vi "zad11.vi"() -> ()   [LabVIEW 2025]
uses:
  state.ctl
  coffee.ctl
  delay_control.ctl
panel:
  out "error out":errorcluster
  in  "error in":errorcluster
  in  "Stop":bool
  out "Whipped cream":bool
  out "Chocolate Syrup":bool
  out "Milk Foam":bool
  out "Steamed Milk":bool
  out "Espresso":bool
  in  "Cafe Mocha":bool
  in  "Cafe Latte":bool
  in  "Espresso Macchiato":bool
  in  "Espresso":bool
  # "Wybierz kawe:"
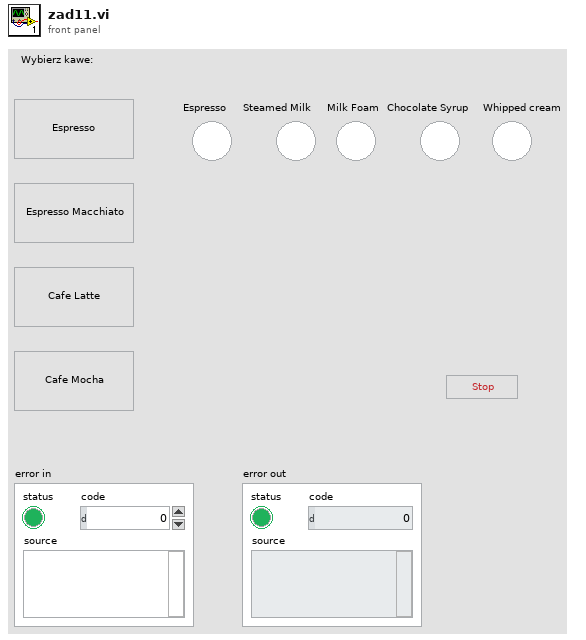
[diagram p1: front panel]
types:
  T1 = typedef "state.ctl" = enum16{"Init", "Idle", "espresso", "milk_foam", "steamed_milk", "whipped_cream", "chocolate_syrup", "save", "stop", "delay"}
  T2 = typedef "delay_control.ctl" = cluster{"time":dbl, "next state":T1}
  T3 = typedef "coffee.ctl" = cluster{"Type_Cof":string, "Cafe":enum16{"None", "espresso", "espresso macchiato", "caffe latte", "cafe mocha"}}
  T4 = enum16{"None", "espresso", "espresso macchiato", "caffe latte", "cafe mocha"}
  T5 = enum16{"open", "replace", "create", "open or create", "replace or create", "replace or create with confirmation"}
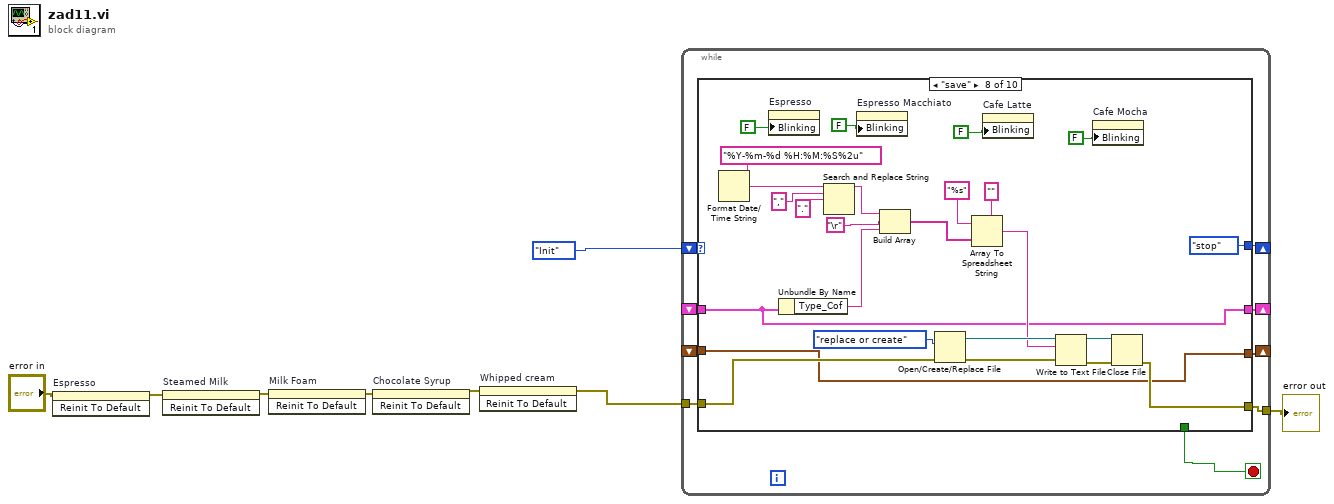
[diagram p0: block diagram]
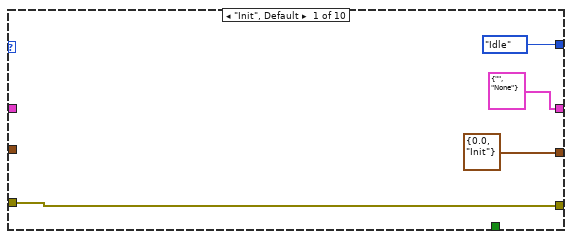
[diagram p2: hidden frame]
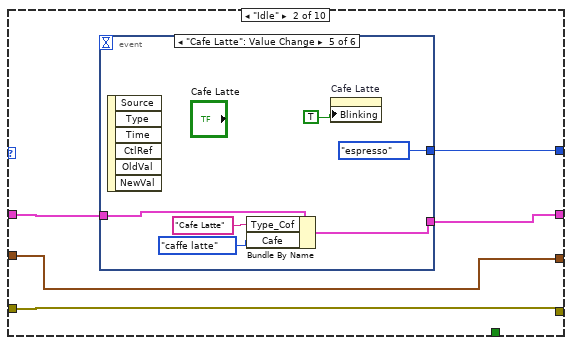
[diagram p3: hidden frame]
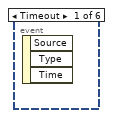
[diagram p4: hidden frame]
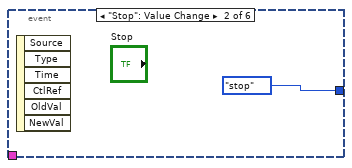
[diagram p5: hidden frame]
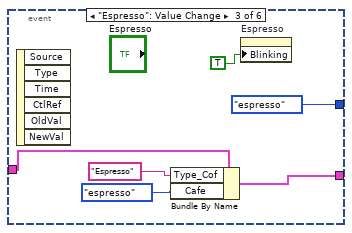
[diagram p6: hidden frame]
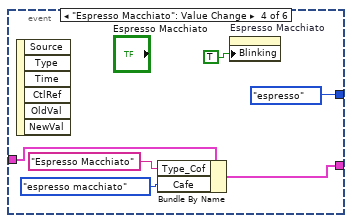
[diagram p7: hidden frame]
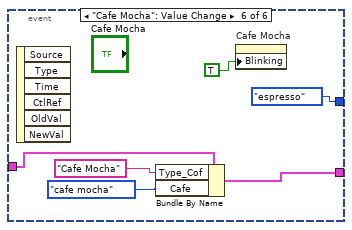
[diagram p8: hidden frame]
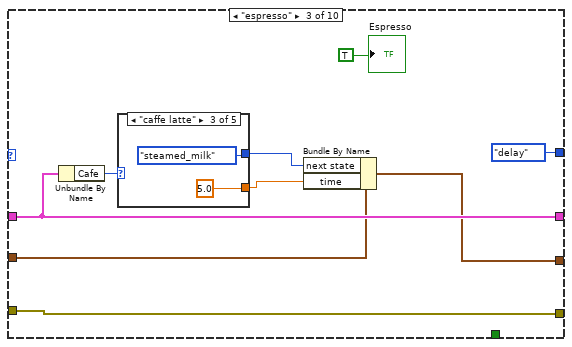
[diagram p9: hidden frame]
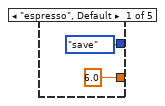
[diagram p10: hidden frame]
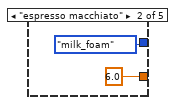
[diagram p11: hidden frame]
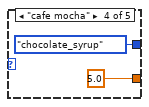
[diagram p12: hidden frame]
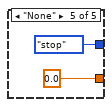
[diagram p13: hidden frame]
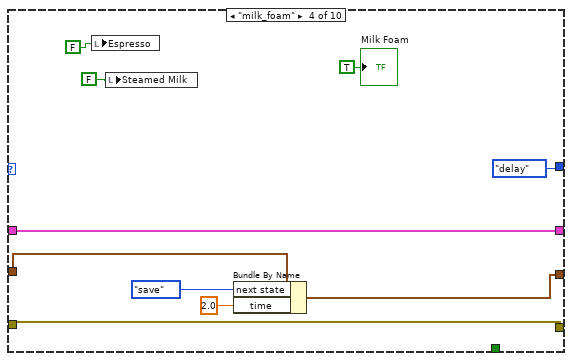
[diagram p14: hidden frame]
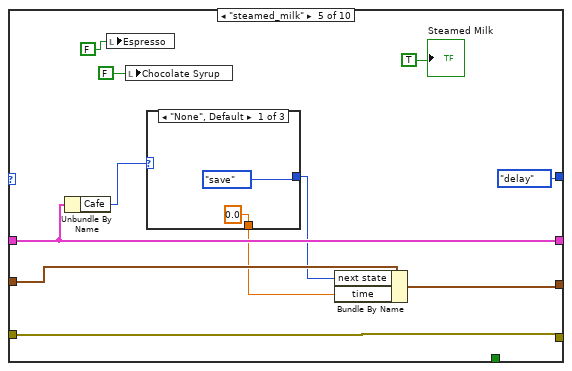
[diagram p15: hidden frame]
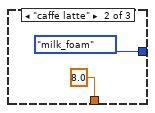
[diagram p16: hidden frame]
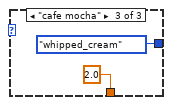
[diagram p17: hidden frame]
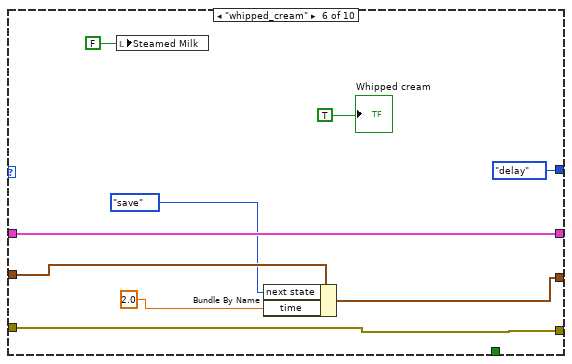
[diagram p18: hidden frame]
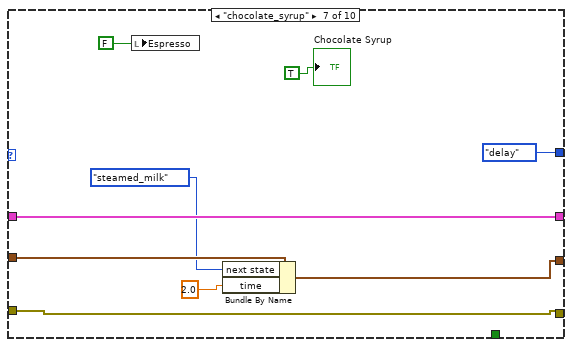
[diagram p19: hidden frame]
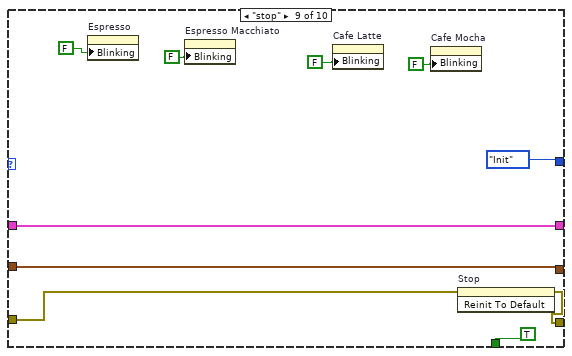
[diagram p20: hidden frame]
diagram:
  n1 = invoke on="Espresso" class="Bool (strict)" method="Reinit To Default"(error in="error in") -> (error out=w2:errorcluster)  [unwired: 2 in, 2 out]
  n2 = invoke on="Steamed Milk" class="Bool (strict)" method="Reinit To Default"(error in=w2) -> (error out=w3:errorcluster)  [unwired: 2 in, 2 out]
  n3 = invoke on="Milk Foam" class="Bool (strict)" method="Reinit To Default"(error in=w3) -> (error out=w4:errorcluster)  [unwired: 2 in, 2 out]
  n4 = invoke on="Chocolate Syrup" class="Bool (strict)" method="Reinit To Default"(error in=w4) -> (error out=w5:errorcluster)  [unwired: 2 in, 2 out]
  n5 = invoke on="Whipped cream" class="Bool (strict)" method="Reinit To Default"(error in=w5) -> (error out=w6:errorcluster)  [unwired: 2 in, 2 out]
  n6 = while {
    tunnel: [w17] -> w8
    tunnel: w6 -> [w16]
    shift-right: [w14] -> _
    shift-left: state."Init" -> [w15]
    shift-right: [w13] -> _
    shift-left: _ -> [w12]
    shift-right: [w10] -> _
    shift-left: _ -> [w9]
    stop <- w11 stop-if-true
    n7 = case shown="\"save\"" w15 {
      tunnel: [w21 w26 w56 w76 w86 w103 w112 w131 w146 w157] -> w17
      tunnel: w16 -> [w21 w26 w56 w76 w86 w103 w112 w134 w145 w157]
      tunnel: [state."Idle" w22 state."delay" state."delay" state."delay" state."delay" state."delay" state."stop" state."Init" w154] -> w14
      tunnel: [T3 {"Type_Cof"="", "Cafe"=enum."None"} w25 w59 w79 w90 w106 w115 w130 w148 w159] -> w13
      tunnel: w12 -> [_ w24 w59 w79 w90 w106 w115 w130 w148 w159]
      tunnel: [_ _ _ _ _ _ _ _ TRUE ("Stop") _] -> w11
      tunnel: [T2 {"time"=0.0, "next state"=enum."Init"} w23 w54 w71 w81 w98 w108 w124 w147 w158] -> w10
      tunnel: w9 -> [_ w23 w55 w75 w85 w101 w111 w124 w147 w158]
      frame "Init", Default {
      }
      frame "Idle" {
        n8 = event shown="[4] \"Cafe Latte\": Value Change" {
          selector: _ -> [_ _ _ _ _ _]
          dyn-events: _ -> [_ _ _ _ _ _]
          timeout: _ -> [_ _ _ _ _ _]
          tunnel: [_ _ w32 w38 w44 w50] -> w25
          tunnel: w24 -> [_ _ w29 w35 w41 w47]
          tunnel: [_ state."stop" state."espresso" state."espresso" state."espresso" state."espresso"] -> w22
          event Timeout {
            n9 = event-data() -> ()  [unwired: 1 in, 3 out]
          }
          event "Stop": Value Change {
            n10 = event-data() -> ()  [unwired: 1 in, 6 out]
          }
          event "Espresso": Value Change {
            n11 = event-data() -> ()  [unwired: 1 in, 6 out]
            n12 = Bundle By Name(cluster=w29, "Type_Cof"="Espresso", "Cafe"=T4."espresso") -> (w32:T3)
            n13 = property on="Espresso" class="Bool"("Blinking"=TRUE) -> ()  [unwired: 2 in, 2 out]
          }
          event "Espresso Macchiato": Value Change {
            n14 = event-data() -> ()  [unwired: 1 in, 6 out]
            n15 = Bundle By Name(cluster=w35, "Type_Cof"="Espresso Macchiato", "Cafe"=T4."espresso macchiato") -> (w38:T3)
            n16 = property on="Espresso Macchiato" class="Bool"("Blinking"=TRUE) -> ()  [unwired: 2 in, 2 out]
          }
          event "Cafe Latte": Value Change {
            n17 = event-data() -> ()  [unwired: 1 in, 6 out]
            n18 = Bundle By Name(cluster=w41, "Type_Cof"="Cafe Latte", "Cafe"=T4."caffe latte") -> (w44:T3)
            n19 = property on="Cafe Latte" class="Bool"("Blinking"=TRUE) -> ()  [unwired: 2 in, 2 out]
          }
          event "Cafe Mocha": Value Change {
            n20 = event-data() -> ()  [unwired: 1 in, 6 out]
            n21 = Bundle By Name(cluster=w47, "Type_Cof"="Cafe Mocha", "Cafe"=T4."cafe mocha" ("Enum")) -> (w50:T3)
            n22 = property on="Cafe Mocha" class="Bool"("Blinking"=TRUE ("Indicator")) -> ()  [unwired: 2 in, 2 out]
          }
        }
      }
      frame "espresso" {
        n23 = Unbundle By Name(w59) -> ("Cafe"=w58:T4)
        n24 = case shown="\"caffe latte\"" w58 {
          tunnel: [6.0 6.0 5.0 5.0 0.0] -> w53
          tunnel: [state."save" state."milk_foam" state."steamed_milk" state."chocolate_syrup" state."stop"] -> w52
          frame "espresso", Default {
          }
          frame "espresso macchiato" {
          }
          frame "caffe latte" {
          }
          frame "cafe mocha" {
          }
          frame "None" {
          }
        }
        n25 = Bundle By Name(cluster=w55, "next state"=w52, "time"=w53) -> (w54:T2)
        "Espresso" <- TRUE ("Espresso")
      }
      frame "milk_foam" {
        n26 = local write "Espresso"(FALSE ("Espresso")) -> ()
        n27 = local write "Steamed Milk"(FALSE ("Steamed Milk")) -> ()
        n28 = Bundle By Name(cluster=w75, "next state"=state."save", "time"=2.0 ("Delay Time (s)")) -> (w71:T2)
        "Milk Foam" <- TRUE ("Milk Foam")
      }
      frame "steamed_milk" {
        n29 = Unbundle By Name(w90) -> ("Cafe"=w89:T4)
        n30 = local write "Espresso"(FALSE ("Espresso")) -> ()
        n31 = local write "Chocolate Syrup"(FALSE ("Chocolate Syrup")) -> ()
        n32 = case shown="\"None\", Default" w89 {
          tunnel: [state."save" state."milk_foam" state."whipped_cream"] -> w83
          tunnel: [0.0 8.0 2.0] -> w82
          frame "None", Default {
          }
          frame "caffe latte" {
          }
          frame "cafe mocha" {
          }
        }
        n33 = Bundle By Name(cluster=w85, "next state"=w83, "time"=w82) -> (w81:T2)
        "Steamed Milk" <- TRUE ("Steamed Milk")
      }
      frame "whipped_cream" {
        n34 = local write "Steamed Milk"(FALSE ("Steamed Milk")) -> ()
        n35 = Bundle By Name(cluster=w101, "next state"=state."save", "time"=2.0 ("Delay Time (s)")) -> (w98:T2)
        "Whipped cream" <- TRUE ("Whipped cream")
      }
      frame "chocolate_syrup" {
        n36 = local write "Espresso"(FALSE ("Espresso")) -> ()
        n37 = Bundle By Name(cluster=w111, "next state"=state."steamed_milk", "time"=2.0 ("Delay Time (s)")) -> (w108:T2)
        "Chocolate Syrup" <- TRUE ("Chocolate Syrup")
      }
      frame "save" {
        n38 = Format Date/Time String(time format string (%c)="%Y-%m-%d %H:%M:%S%2u") -> (date/time string=w120:string)  [unwired: 2 in]
        n39 = property on="Espresso" class="Bool"("Blinking"=FALSE) -> ()  [unwired: 2 in, 2 out]
        n40 = Unbundle By Name(w130) -> ("Type_Cof"=w118:string)
        n41 = Search and Replace String(input string=w120, search string=",", replace string="." ("replace string (\"\")")) -> (result string=w119:string)  [unwired: 5 in, 3 out]
        n42 = property on="Espresso Macchiato" class="Bool"("Blinking"=FALSE) -> ()  [unwired: 2 in, 2 out]
        n43 = Build Array(w119, "\r", w118) -> (w139:string[])
        n44 = Open/Create/Replace File(error in=w134, operation (0:open)=T5."replace or create") -> (refnum out=w137:refnum<file>, error out=w133:errorcluster)  [unwired: 4 in, 1 out]
        n45 = Array To Spreadsheet String(delimiter (Tab)="", array=w139, 3:"%s" ("format string")) -> (spreadsheet string=w135:string)
        n46 = property on="Cafe Latte" class="Bool"("Blinking"=FALSE) -> ()  [unwired: 2 in, 2 out]
        n47 = Write to Text File(file (use dialog)=w137, text=w135, error in=w133) -> (refnum out=w136:refnum<file>, error out=w132:errorcluster)  [unwired: 1 in, 1 out]
        n48 = property on="Cafe Mocha" class="Bool"("Blinking"=FALSE) -> ()  [unwired: 2 in, 2 out]
        n49 = Close File(refnum=w136, error in=w132) -> (error out=w131:errorcluster)  [unwired: 1 out]
      }
      frame "stop" {
        n50 = property on="Espresso" class="Bool"("Blinking"=FALSE) -> ()  [unwired: 2 in, 2 out]
        n51 = property on="Espresso Macchiato" class="Bool"("Blinking"=FALSE) -> ()  [unwired: 2 in, 2 out]
        n52 = property on="Cafe Latte" class="Bool"("Blinking"=FALSE) -> ()  [unwired: 2 in, 2 out]
        n53 = property on="Cafe Mocha" class="Bool"("Blinking"=FALSE) -> ()  [unwired: 2 in, 2 out]
        n54 = invoke on="Stop" class="Bool" method="Reinit To Default"(error in=w145) -> (error out=w146:errorcluster)  [unwired: 2 in, 2 out]
      }
      frame "delay" {
        n55 = Unbundle By Name(w158) -> ("time"=w152:dbl, "next state"=w153:T1)
        n56 = Multiply(x=1000.0 ("y"), y=w152) -> (x*y=w156:dbl)
        n57 = To Long Integer(number=w156) -> (32bit integer=w155:i32)
        n58 = event shown="[1] \"Stop\": Value Change" {
          selector: _ -> [_ _]
          dyn-events: _ -> [_ _]
          timeout: w155 -> [_ _]
          tunnel: [w160 state."stop"] -> w154
          tunnel: w153 -> [w160 _]
          event Timeout {
            n59 = event-data() -> ()  [unwired: 1 in, 3 out]
          }
          event "Stop": Value Change {
            n60 = event-data() -> ()  [unwired: 1 in, 3 out]
          }
        }
      }
    }
  }
  "error out" <- w8
